vi "PROJECT_SplashScreen.vi"(11 "Show only static About info":bool) -> ()   [LabVIEW 2020, in "Project.lvlib"]
doc: "____\nHAMPEL SOFTWARE ENGINEERING v2.6.0 (2023-12-19 10:54)"
uses:
  Project.lvlib
  Libraries/hse-libraries/Source/hse-ui/Screens/Screen_Event.ctl
  Libraries/hse-libraries/Source/hse-application/hse-application.lvclass/hse-application.ctl
  Libraries/hse-libraries/Source/hse-application/HSE Application not initialized--error.vi
  <vilib>/Utility/error.llb/Clear Errors.vi
  Libraries/hse-libraries/Source/hse-application/hse-application__GetSingleton.vi
  <vilib>/Utility/error.llb/Error Cluster From Error Code.vi
  <vilib>/Utility/cursorutil.llb/Set Cursor (Icon Pict).vi
  <vilib>/Platform/browser.llb/Open URL in Default Browser (string).vi
  Libraries/hse-libraries/Source/hse-ui/hse-ui.lvlib
  Libraries/hse-libraries/Source/hse-application/hse-application.lvclass
panel:
  in  "Continue Startup UE":refnum<user-event>
  in  "Btn_Website":bool
  in  "Btn_Close":bool
  out "Copyright Notices":string
  out "HSE Libraries Version:":string
  out "HSE Framework Version:":string
  out "Application Version:":string
  out "Application Name:":string
  out "String":string
  out "Slide":u8(slide) scale=0.0..100.0
  in  "Splash VI Event":refnum<user-event>
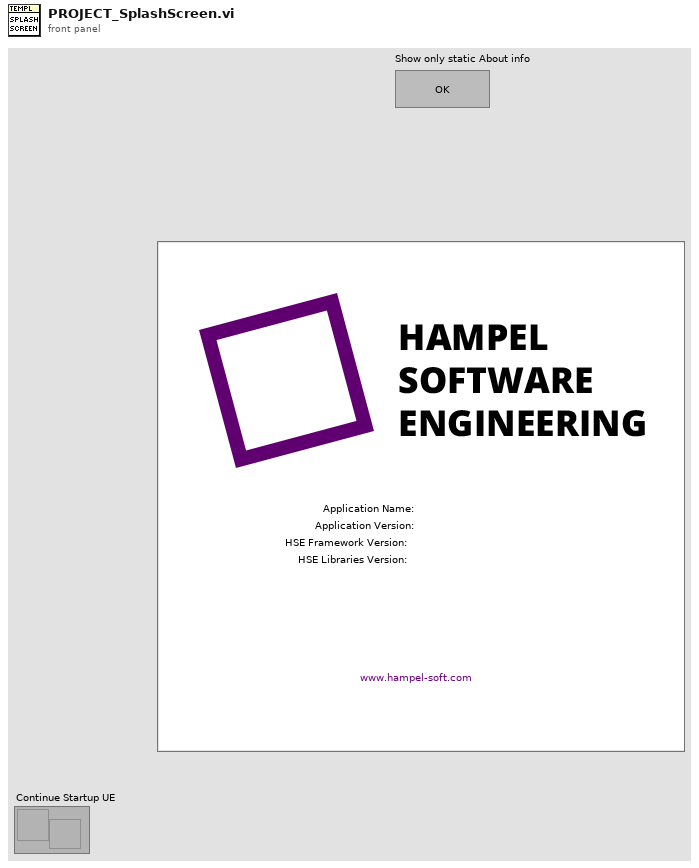
[diagram p1: front panel]
types:
  T1 = enum32{"Invalid", "Standard", "Closed", "Hidden", "Minimized", "Maximized"}
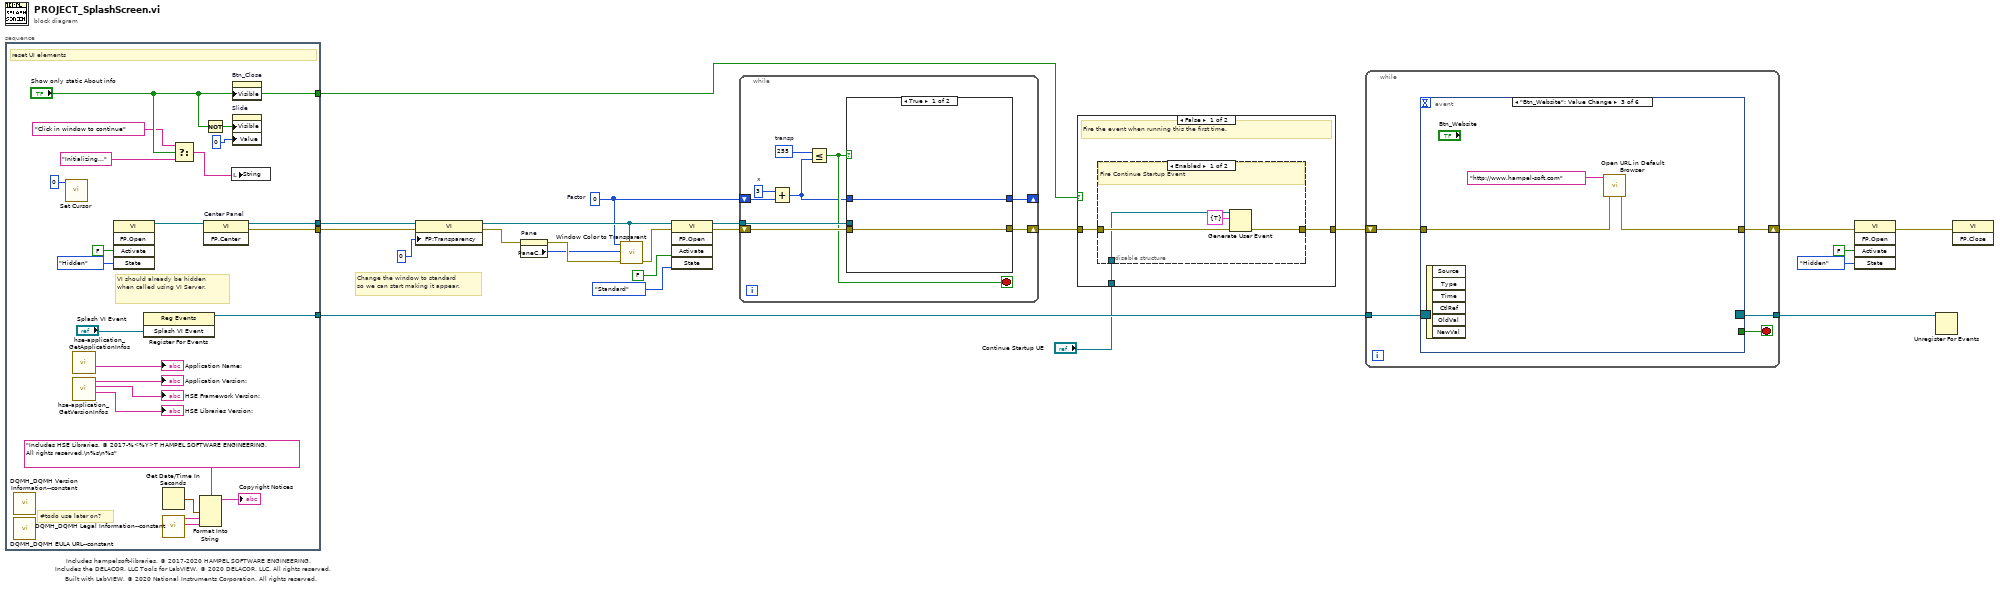
[diagram p0: block diagram]
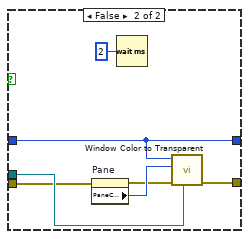
[diagram p4: hidden frame]
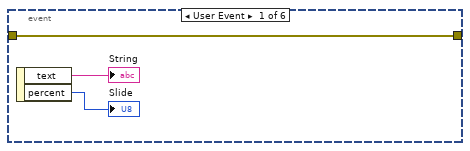
[diagram p5: hidden frame]
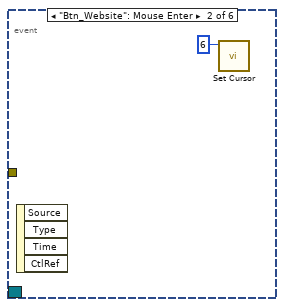
[diagram p6: hidden frame]
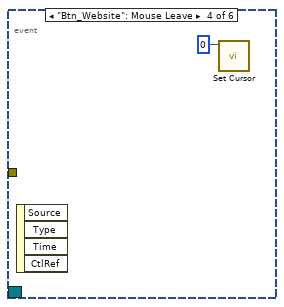
[diagram p7: hidden frame]
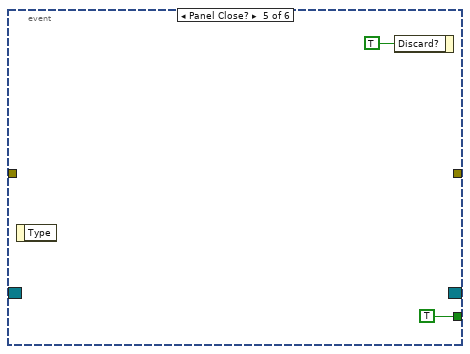
[diagram p8: hidden frame]
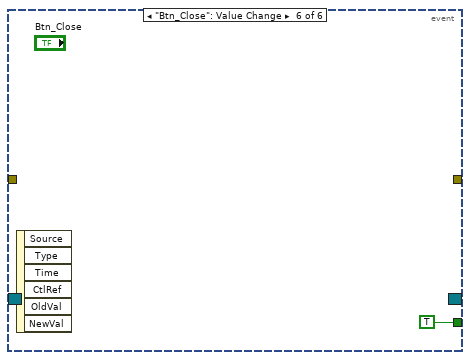
[diagram p9: hidden frame]
diagram:
  w9 = u8 0  # Factor
  # "Built with LabVIEW, © 2020 National Instruments Corporation. All rights reserved."
  # "Includes the DELACOR, LLC Tools for LabVIEW, © 2020 DELACOR, LLC. All rights reserved."
  # "Includes hampelsoft-libraries, © 2017-2020 HAMPEL SOFTWARE ENGINEERING."
  # "Change the window to standard\nso we can start making it appear."
  n1 = stacked-sequence {
    tunnel: [w41] -> w21
    tunnel: [w40] -> w20
    tunnel: [w43] -> w22
    tunnel: ["Show only static About info"] -> w1
    frame #0 {
      # "#todo use later on?"
      # "VI should already be hidden when called using VI Server."
      # "reset UI elements"
      n2 = call <vilib>:"DQMH_DQMH Version Information--constant.vi"() -> ()  [unwired: 11 in, 1 out]
      n3 = call <vilib>:"DQMH_DQMH EULA URL--constant.vi"() -> ()  [unwired: 11 in, 1 out]
      n4 = call-poly <vilib>:"Set Cursor.vi"("icon"=u16 0) -> ()  [unwired: 9 in, 2 out]
      n5 = call "hse-application_GetApplicationInfos.vi"() -> ("Application Name"=→"Application Name:":string)  [unwired: 8 in, 3 out]
      n6 = call "hse-application_GetVersionInfos.vi"() -> ("HSE-LIB Version"=→"HSE Libraries Version:":string, "Framework Version"=→"HSE Framework Version:":string, "Application Version"=→"Application Version:":string)  [unwired: 6 in, 3 out]
      n7 = invoke class="VI" method="FP.Open"("Activate"=FALSE ("Activate?"), "State"=T1."Hidden") -> (reference out=w42:refnum<vi>)  [unwired: 3 in, 4 out]
      n8 = register-events("Splash VI Event") -> (reference out=w43:refnum<event-registration>)  [unwired: 2 in, 1 out]
      n9 = Get Date/Time In Seconds() -> (seconds since 1Jan1904=w24:timestamp)
      n10 = call <vilib>:"DQMH_DQMH Legal Information--constant.vi"() -> ("LabVIEW Legal"=w26:string, "DQMH Legal"=w27:string)  [unwired: 10 in]
      n11 = Select(t="Click in window to continue", s="Show only static About info", f="Initializing...") -> (s? t:f=w34:string)
      n12 = Format Into String(format string="Includes HSE Libraries, © 2017-%<%Y>T HAMPEL SOFTWARE ENGINEERING. All rights reserved.\n%s\n%s", w24, w27, w26) -> (resulting string=→"Copyright Notices":string)  [unwired: 2 in, 1 out]
      n13 = invoke on="Center Panel" class="VI" method="FP.Center"(reference=w42) -> (reference out=w41:refnum<vi>, error out=w40:errorcluster)  [unwired: 2 in, 1 out]
      n14 = Not(x="Show only static About info") -> (.not. x?=w39:bool)
      n15 = local write "String"(w34) -> ()
      n16 = property on="Btn_Close" class="Bool"("Visible"="Show only static About info") -> ()  [unwired: 2 in, 2 out]
      n17 = property on="Slide" class="Slide (strict)"("Visible"=w39, "Value"=u8 0 ("Slide")) -> ()  [unwired: 2 in, 2 out]
    }
  }
  n18 = property class="VI"(reference=w21, error in=w20, "FP:Transparency"=u8 0 ("t")) -> (reference out=w11:refnum<vi>, error out=w13:errorcluster)
  n19 = property on="Pane" class="Pane"(error in=w13) -> (error out=w17:errorcluster, "PaneColor"=w16:u32)  [unwired: 1 in, 1 out]
  n20 = call "Window Color to Transparent.vi"("Calling VI's reference"=w11, "error in (no error)"=w17, "Color to Replace"=w16, "Factor"=w9) -> ("error out"=w12:errorcluster)  [unwired: 7 in]
  n21 = invoke class="VI" method="FP.Open"(reference=w11, error in=w12, "Activate"=FALSE ("Activate?"), "State"=T1."Standard") -> (reference out=w15:refnum<vi>, error out=w14:errorcluster)  [unwired: 1 in, 3 out]
  n22 = while {
    shift-right: [w53] -> _
    shift-left: w9 -> [w49]
    shift-right: [w52] -> w4
    shift-left: w14 -> [w51]
    tunnel: w15 -> [w54]
    stop <- w50 stop-if-true
    w47 = u8 3  # x
    w55 = u8 255  # transp
    n23 = Add(x=w47, y=w49) -> (x+y=w48:u8)
    n24 = Less Or Equal?(x=w55, y=w48) -> (x <= y?=w50:bool)
    n25 = case shown="True" w50 {
      tunnel: w48 -> [w57 w61]
      tunnel: w54 -> [_ w62]
      tunnel: [w57 w61] -> w53
      tunnel: [w56 w60] -> w52
      tunnel: w51 -> [w56 w59]
      frame True {
      }
      frame False {
        n26 = property on="Pane" class="Pane"(error in=w59) -> (error out=w63:errorcluster, "PaneColor"=w64:u32)  [unwired: 1 in, 1 out]
        n27 = Wait (ms)(milliseconds to wait=u32 2) -> ()  [unwired: 1 out]
        n28 = call "Window Color to Transparent.vi"("Calling VI's reference"=w62, "error in (no error)"=w63, "Color to Replace"=w64, "Factor"=w61) -> ("error out"=w60:errorcluster)  [unwired: 7 in]
      }
    }
  }
  n29 = case shown="False" w1 {
    tunnel: w4 -> [w67 w73]
    tunnel: [w66 w73] -> w3
    tunnel: "Continue Startup UE" -> [w65 _]
    frame False {
      # "Fire the event when running this the first time."
      n30 = disable-structure shown="Enabled" {
        disable-tunnel: w67 -> [w71 w72]
        disable-tunnel: [w70 w72] -> w66
        disable-tunnel: w65 -> [w69 _]
        frame Enabled {
          # "Fire Continue Startup Event"
          n31 = Generate User Event(user event=w69, event data cluster=cluster{"Continue Startup":bool} {"Continue Startup"=TRUE} ("event data"), error in=w71) -> (error out=w70:errorcluster)  [unwired: 1 in, 1 out]
        }
        frame Disabled {
          # "Implement your code here."
        }
      }
    }
    frame True {
      # "Do not fire the event if Splash VI called from running application."
    }
  }
  n32 = while {
    shift-right: [w78] -> w6
    shift-left: w3 -> [w76]
    tunnel: [w75] -> w23
    tunnel: w22 -> [w74]
    stop <- w77 stop-if-true
    n33 = event shown="[2] \"Btn_Website\": Value Change" {
      selector: w74 -> [_ _ _ _ _ _]
      dyn-events: [_ _ _ _ _ _] -> w75
      timeout: _ -> [_ _ _ _ _ _]
      tunnel: w76 -> [w81 _ w83 _ _ _]
      tunnel: [w81 _ w84 _ _ _] -> w78
      tunnel: [_ _ _ _ TRUE ("Close") TRUE ("Close")] -> w77
      event User Event {
        n34 = event-data() -> ("text"=→"String":string, "percent"=→"Slide":i32)  [unwired: 1 in]
      }
      event "Btn_Website": Mouse Enter {
        n35 = event-data() -> ()  [unwired: 1 in, 4 out]
        n36 = call-poly <vilib>:"Set Cursor.vi"("icon"=u16 6) -> ()  [unwired: 9 in, 2 out]
      }
      event "Btn_Website": Value Change {
        n37 = event-data() -> ()  [unwired: 1 in, 6 out]
        n38 = call-poly <vilib>:"Open URL in Default Browser.vi"("error in (no error)"=w83, "URL"="http://www.hampel-soft.com" ("Link")) -> ("error out"=w84:errorcluster)  [unwired: 4 in, 1 out]
      }
      event "Btn_Website": Mouse Leave {
        n39 = event-data() -> ()  [unwired: 1 in, 4 out]
        n40 = call-poly <vilib>:"Set Cursor.vi"("icon"=u16 0) -> ()  [unwired: 9 in, 2 out]
      }
      event Panel Close? {
        n41 = event-data() -> ()  [unwired: 1 in, 1 out]
        n42 = event-data("Discard?"=TRUE) -> ()  [unwired: 1 in, 1 out]
      }
      event "Btn_Close": Value Change {
        n43 = event-data() -> ()  [unwired: 1 in, 6 out]
      }
    }
  }
  n44 = invoke class="VI" method="FP.Open"(error in=w6, "Activate"=FALSE ("Activate?"), "State"=T1."Hidden") -> (error out=w5:errorcluster)  [unwired: 2 in, 4 out]
  n45 = Unregister For Events(event registration refnum=w23) -> ()  [unwired: 1 in, 1 out]
  n46 = invoke class="VI" method="FP.Close"(error in=w5) -> ()  [unwired: 2 in, 3 out]
